vi "SETTING CLOSE GLOBEL VARIABLE.vi"() -> ()   [LabVIEW 2021]
panel:
  out "SETTINGS CLOSE":bool
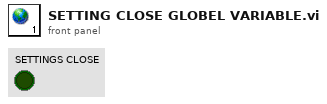
[diagram p1: front panel]
diagram:
